vi "AMX-SaveImage - 衬丝检测.vi"(0 "基路径":path, 1 "CCD Name":string(combo), 5 "布尔":bool=TRUE, 7 "结果":bool=TRUE, 9 "Image in":T1(plugin-control), 11 "error in (no error)":errorcluster) -> (15 "error out":errorcluster)   [LabVIEW 2017]
panel:
  out "连接的字符串":string
  # "D:\\Data\\History Image\\20190228\\CCD3\\Image"
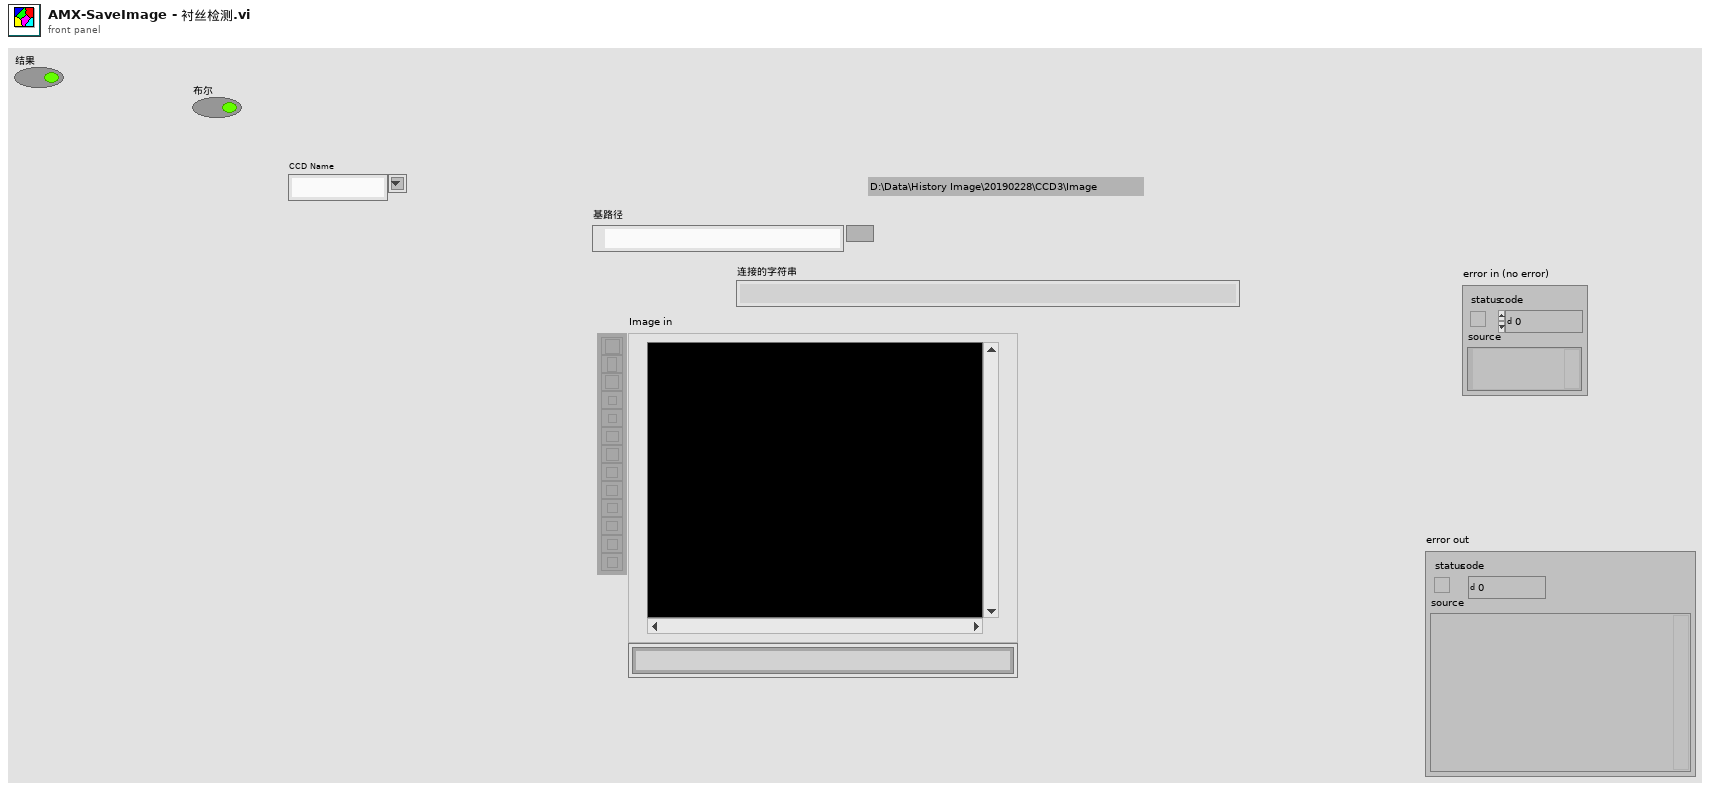
[diagram p1: front panel]
types:
  T1 = typedef "IMAQ Image.ctl" = refnum<image>
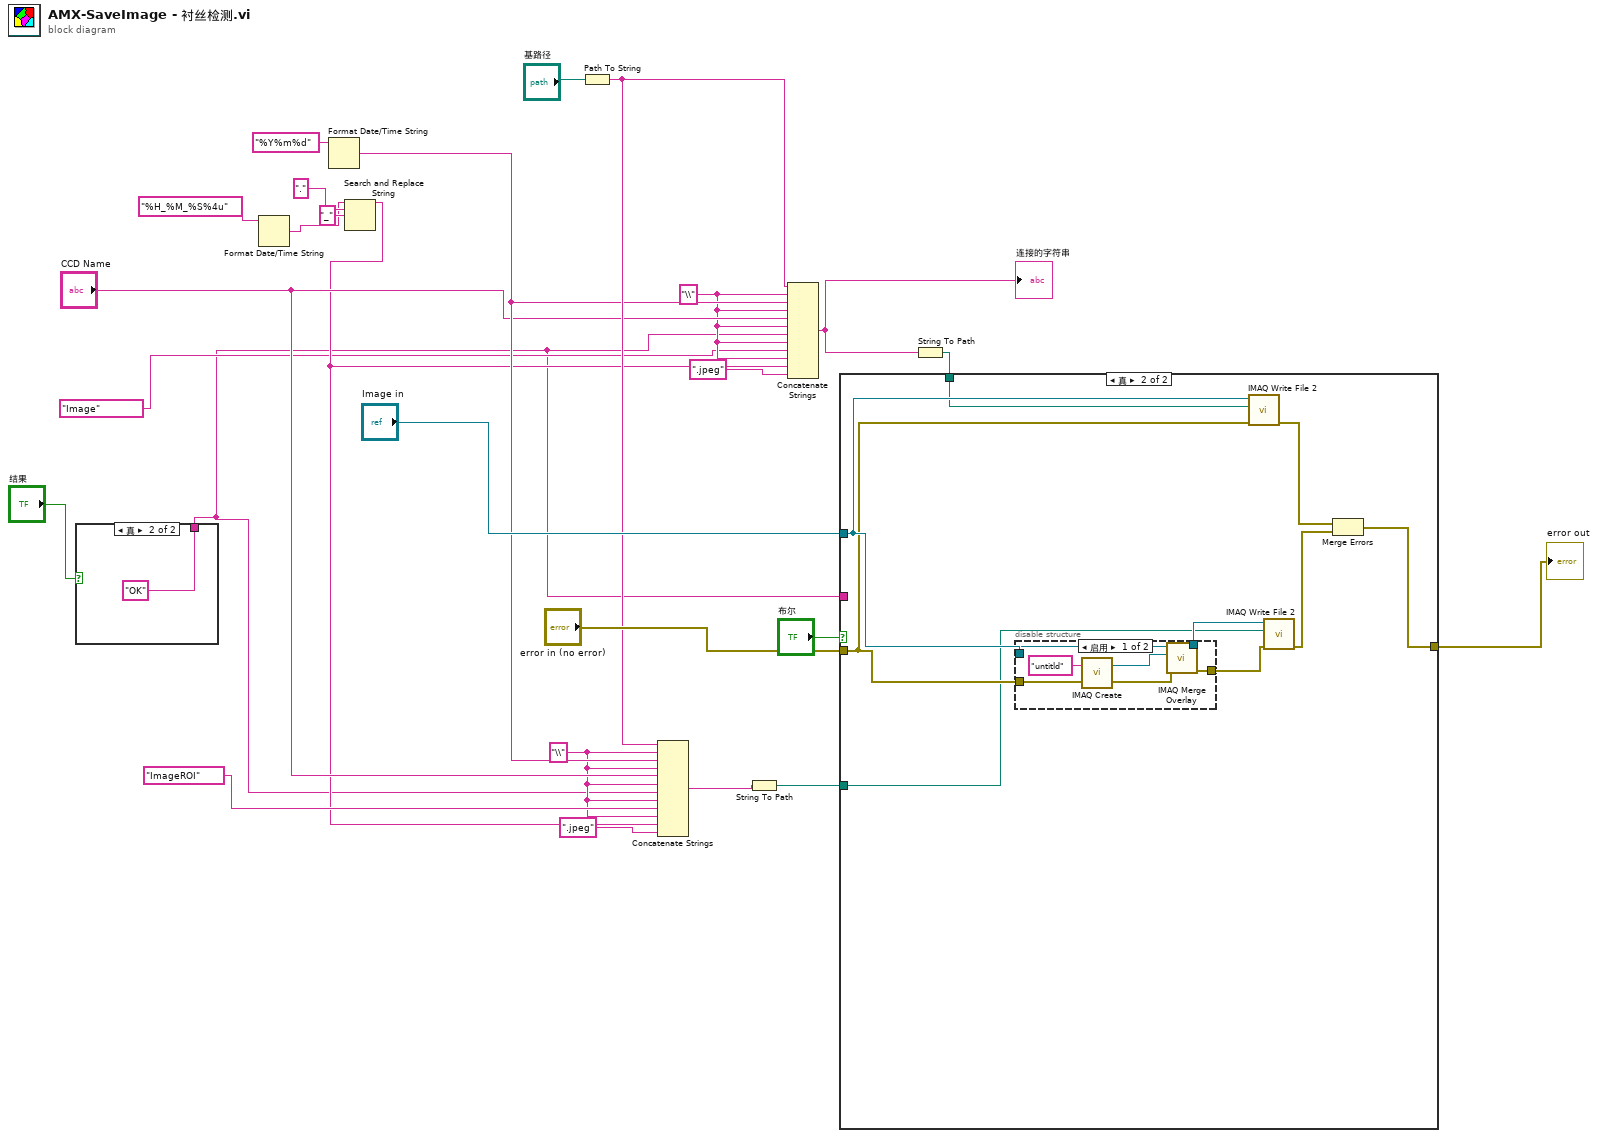
[diagram p0: block diagram]
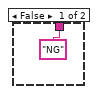
[diagram p2: hidden frame]
diagram:
  w2 = "\\" ("字符串")
  w4 = "\\" ("字符串")
  n1 = case shown="真" "结果" {
    tunnel: ["NG" "OK"] -> w1
    frame False {
    }
    frame True {
    }
  }
  n2 = Format Date/Time String(time format string (%c)="%H_%M_%S%4u" ("时间格式字符串(%c)")) -> (date/time string=w7:string)  [unwired: 2 in]
  n3 = Format Date/Time String(time format string (%c)="%Y%m%d" ("时间格式字符串(%c)")) -> (date/time string=w14:string)  [unwired: 2 in]
  n4 = Search and Replace String(input string=w7, search string="." ("搜索字符串"), replace string="_" ("替换字符串(\"\")")) -> (result string=w6:string)  [unwired: 5 in, 3 out]
  n5 = Path To String(path="基路径") -> (string=w15:string)
  n6 = Concatenate Strings(w15, w2, w14, w2, "CCD Name", w2, w1, w2, "ImageROI" ("类型"), w2, w6, ".jpeg" ("字符串")) -> (w11:string)
  n7 = String To Path(string=w11) -> (path=w10:path)
  n8 = Concatenate Strings(w15, w4, w14, w4, "CCD Name", w4, w1, w4, "Image" ("类型"), w4, w6, ".jpeg" ("字符串")) -> (w24:string)
  "连接的字符串" <- w24
  n9 = String To Path(string=w24) -> (path=w20:path)
  n10 = case shown="真" "布尔" {
    tunnel: "Image in" -> [_ w38]
    tunnel: "error in (no error)" -> [w29 w37]
    tunnel: w20 -> [_ w31]
    tunnel: [w29 w30] -> w18
    tunnel: w1 -> [_ _]
    tunnel: w10 -> [_ w32]
    frame False {
    }
    frame True {
      n11 = disable-structure shown="启用" {
        disable-tunnel: w38 -> [w45 w46]
        disable-tunnel: w37 -> [w44 _]
        disable-tunnel: [w43 w46] -> w36
        disable-tunnel: [w42 _] -> w35
        frame Enabled {
          n12 = call "IMAQ Create"("Image Name"="untitld", "error in (no error)"=w44) -> ("New Image"=w40:T1, "error out"=w39:errorcluster)  [unwired: 3 in]
          n13 = call "IMAQ Merge Overlay"("error in (no error)"=w39, "Image Dst"=w40, "Image Src"=w45) -> ("error out"=w42:errorcluster, "Image Dst Out"=w43:T1)  [unwired: 7 in]
        }
        frame Disabled {
        }
      }
      n14 = call-poly "IMAQ Write File 2"("error in (no error)"=w37, "File Path"=w31, "Image"=w38) -> ("error out"=w33:errorcluster)  [unwired: 7 in, 1 out]
      n15 = call-poly "IMAQ Write File 2"("error in (no error)"=w35, "File Path"=w32, "Image"=w36) -> ("error out"=w34:errorcluster)  [unwired: 7 in, 1 out]
      n16 = Merge Errors(w33, w34) -> (w30:errorcluster)
    }
  }
  "error out" <- w18
